vi "RisingEdgeDetect.vi"(1 "Input":bool) -> (0 "Output":bool)   [LabVIEW 2013]
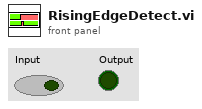
[diagram p1: front panel]
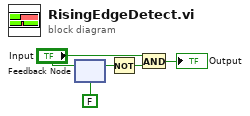
[diagram p0: block diagram]
diagram:
  n1 = feedback #1(FALSE) -> (w1:bool)
  n2 = feedback-in #1("Input") -> ()
  n3 = Not(x=w1) -> (.not. x?=w2:bool)
  n4 = And(x="Input", y=w2) -> (x .and. y?=→"Output":bool)
